vi "testSelectState(s)SimpleFalse_Boolean.vi"(8 "error in (no error)":errorcluster, 11 "testStateMachineUtilities in":refnum<class "testStateMachineUtilities.lvclass">) -> (0 "error out":errorcluster, 3 "testStateMachineUtilities out":refnum<class "testStateMachineUtilities.lvclass">)   [LabVIEW 2013, in "testStateMachineUtilities.lvclass"]
uses:
  testStateMachineUtilities.lvclass
  source/State Machine Support API/Select State(s)_bool.vi
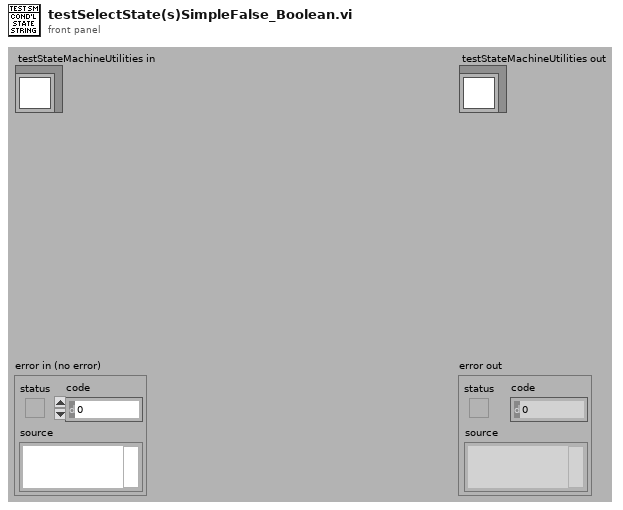
[diagram p1: front panel]
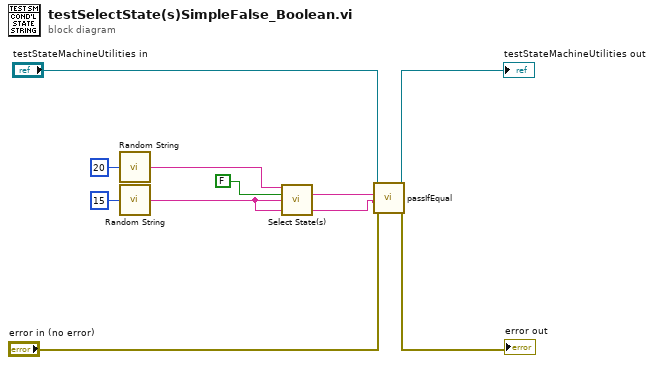
[diagram p0: block diagram]
diagram:
  n1 = call "Random String.vi"("Length"=20) -> ("ASCII"=w2:string)  [unwired: 4 in]
  n2 = call "Random String.vi"("Length"=15) -> ("ASCII"=w1:string)  [unwired: 4 in]
  n3 = call-poly "Select State(s).vi"("State(s) if True (\"\")"=w2, "Select"=FALSE ("Do State(s)?"), "State(s) if False (\"\")"=w1) -> ("States Out"=w3:string)  [unwired: 12 in]
  n4 = call-dynamic "passIfEqual.vi"("error in (no error)"="error in (no error)", "y"=w1, "x"=w3, "TestCase in"="testStateMachineUtilities in") -> ("error out"=→"error out":errorcluster, "TestCase out"=→"testStateMachineUtilities out":refnum<class "testStateMachineUtilities.lvclass">)  [unwired: 6 in]
